vi "video.update_add_label.vi"(8 "error in":errorcluster, 11 "VideoUpdateStaging in":refnum<class "VideoUpdateStaging.lvclass">) -> (0 "error out":errorcluster, 3 "VideoUpdateStaging out":refnum<class "VideoUpdateStaging.lvclass">)   [LabVIEW 2020, in "VideoUpdateStaging.lvclass"]
doc: "Adds a label to the set of labels that will replace the video's current labels."
uses:
  VideoUpdateStaging.lvclass
  VideoUpdateStaging.lvclass/VideoUpdateStaging.ctl
  client.lvlib
panel:
  in  "label":string
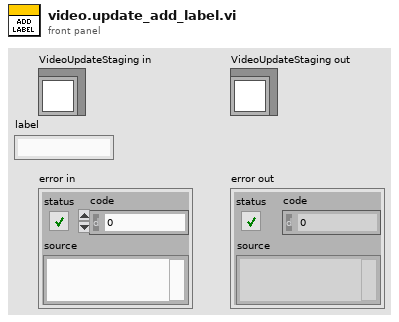
[diagram p1: front panel]
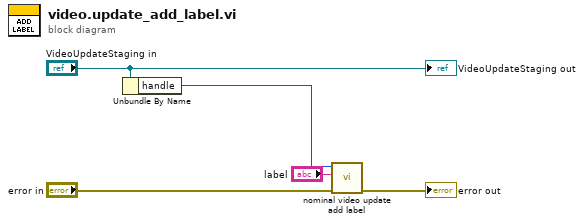
[diagram p0: block diagram]
diagram:
  n1 = Unbundle By Name("VideoUpdateStaging in") -> ("handle"=w3:i32)
  n2 = call "nominal video update add label.vi"("error in (no error)"="error in", "label"="label", "staging"=w3) -> ("error out"=→"error out":errorcluster)  [unwired: 7 in, 1 out]
  "VideoUpdateStaging out" <- "VideoUpdateStaging in"
